vi "DigitalOscilloscope.vi"() -> ()   [LabVIEW 2015]
panel:
  in  "Digitizing Parameters":T1
  out "Waveform Graph":dbl[](graph)
  in  "stop":bool
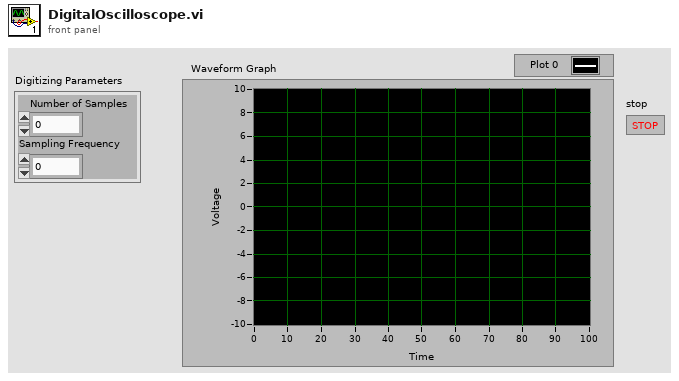
[diagram p1: front panel]
types:
  T1 = cluster{"Number of Samples":i32, "Sampling Frequency":i32}
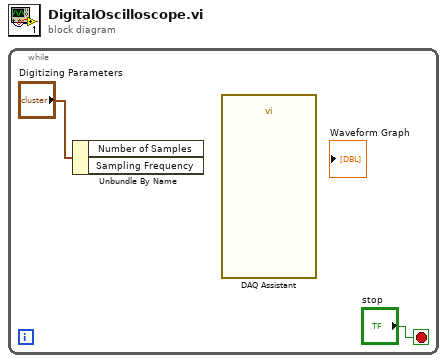
[diagram p0: block diagram]
diagram:
  n1 = while {
    stop <- "stop" stop-if-true
    n2 = Unbundle By Name("Digitizing Parameters") -> ()  [unwired: 2 out]
    n3 = call "DAQ Assistant"() -> ()  [unwired: 17 in, 3 out]
  }
